vi "RTD to Temp (1000Ohms - NI9226).vi"(2 "C":dbl=-4.182999866625403e-12 format="%0.5e", 3 "B":dbl=-5.774199962615967e-07, 4 "A":dbl=0.003908019978553057 format="%0.5e", 5 "RTD Resistance":dbl=0.014999999664723873 format="%.5f") -> (0 "Coeff Out of Range":bool, 1 "RTDtemp":dbl format="%.6f")   [LabVIEW 2018]
uses:
  <vilib>/Analysis/polynomials.llb/Polynomial Roots (DBL).vi
  <vilib>/Analysis/NI_AALPro.lvlib
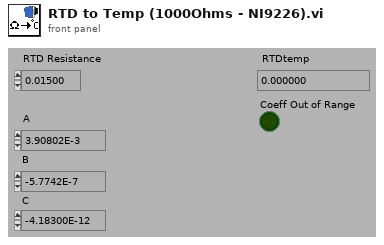
[diagram p1: front panel]
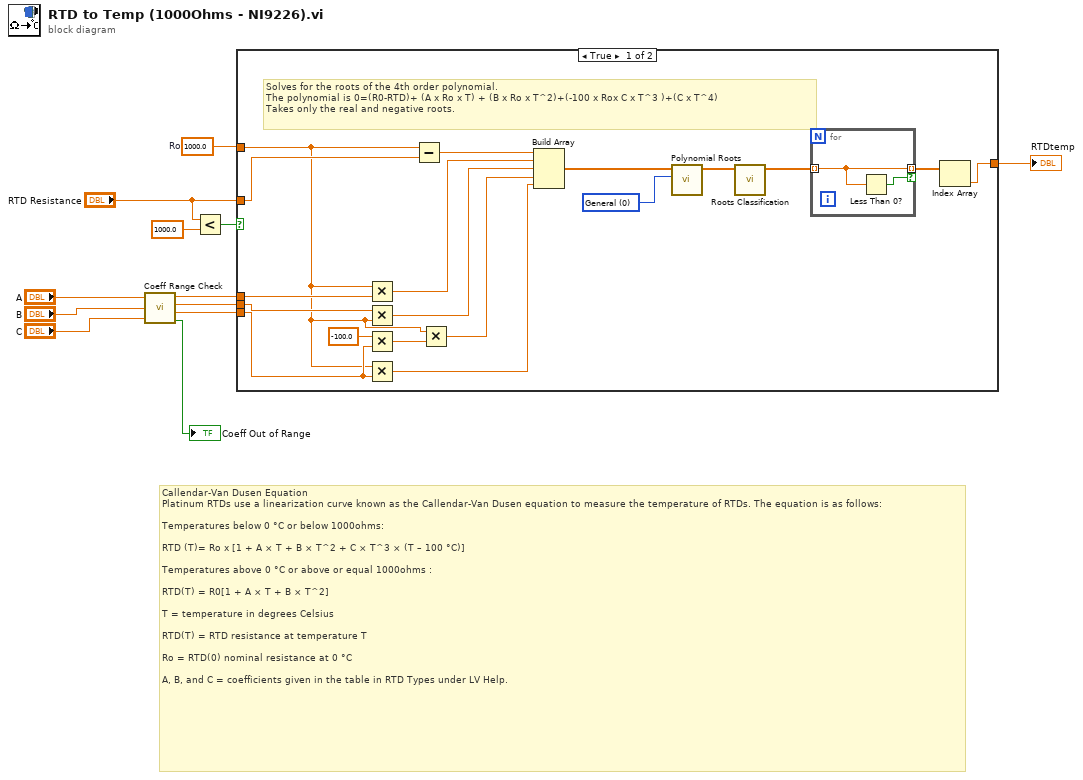
[diagram p0: block diagram]
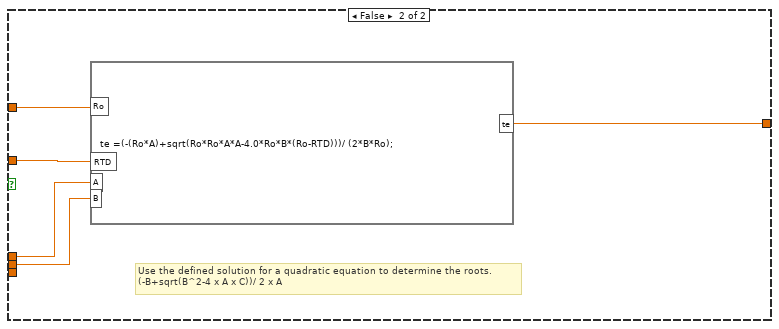
[diagram p2: hidden frame]
diagram:
  w8 = 1000.0  # Ro
  # "Callendar-Van Dusen Equation\nPlatinum RTDs use a linearization curve known as the Callendar-Van Dusen equation to measure the temperature of RTDs. The equation is as follows:\n\nTemperatures below 0 °C or below 1000ohms:\n\nRTD (T)= Ro x [1 + A × T + B × T^2 + C × T^3 × (T – 100 °C)]\n\nTemperatures above 0 °C or above or equal 1000ohms :\n\nRTD(T) = R0[1 + A × T + B × T^2]\n\nT = temperature in degrees Celsius\n\nRTD(T) = RTD resistance at temperature T\n\nRo = RTD(0) nominal resistance at 0 °C\n\nA, B, and C = coefficients given in the table in RTD Types under LV Help."
  n1 = call "Coeff Range Check.vi"("A"="A", "B"="B", "C"="C") -> ("A"=w7:dbl, "B"=w6:dbl, "C"=w5:dbl, "Coeff Out of Range"=→"Coeff Out of Range":bool)
  n2 = Less?(x="RTD Resistance", y=1000.0) -> (x < y?=w11:bool)
  n3 = case shown="True" w11 {
    tunnel: "RTD Resistance" -> [w28 w37]
    tunnel: w6 -> [w23 w36]
    tunnel: w7 -> [w26 w35]
    tunnel: w8 -> [w13 w34]
    tunnel: [w15 w33] -> w12
    tunnel: w5 -> [w18 _]
    frame True {
      w30 = u16 0 items=["General", "Simple Classification", "Refinement", "Advanced Refinement"] ("option")
      # "Solves for the roots of the 4th order polynomial. \nThe polynomial is 0=(R0-RTD)+ (A x Ro x T) + (B x Ro x T^2)+(-100 x Rox C x T^3 )+(C x T^4)\nTakes only the real and negative roots."
      n4 = Multiply(x=w13, y=w26) -> (x*y=w25:dbl)
      n5 = Multiply(x=w23, y=w13) -> (x*y=w22:dbl)
      n6 = Multiply(x=-100.0, y=w18) -> (x*y=w20:dbl)
      n7 = Multiply(x=w13, y=w18) -> (x*y=w21:dbl)
      n8 = Subtract(x=w13, y=w28) -> (x-y=w27:dbl)
      n9 = Multiply(x=w13, y=w20) -> (x*y=w14:dbl)
      n10 = Build Array(w27, w25, w22, w14, w21) -> (w24:dbl[])
      n11 = call-poly <vilib>:"Polynomial Roots.vi"("option"=w30, "P(x)"=w24) -> ("Roots"=w29:cdb[])  [unwired: 8 in, 1 out]
      n12 = call <vilib>:"Roots Classification.vi"("Roots"=w29) -> ("Real Roots"=w17:dbl[])  [unwired: 7 in, 3 out]
      n13 = for {
        tunnel: [w31] -> w16 mode=indexing if=w32
        tunnel: w17 -> [w31] mode=indexing
        n14 = Less Than 0?(x=w31) -> (x < 0?=w32:bool)
      }
      n15 = Index Array(array=w16) -> (element=w15:dbl)  [unwired: 1 in]
    }
    frame False {
      # "Use the defined solution for a quadratic equation to determine the roots.\n(-B+sqrt(B^2-4 x A x C))/ 2 x A"
      n16 = formula code="te =(-(Ro*A)+sqrt(Ro*Ro*A*A-4.0*Ro*B*(Ro-RTD)))/ (2*B*Ro);" ("DEFAULT RTD CONVERSION")("RTD"=w37, "Ro"=w34, "A"=w35, "B"=w36) -> ("te"=w33:dbl)
    }
  }
  "RTDtemp" <- w12
